vi "Clone.vi"(8 "Error In":errorcluster, 11 "reference in":refnum<class "Rectangle.lvclass">) -> (0 "Error Out":errorcluster, 2 "Return(LabVIEW Object)":refnum<class "ICloneable.lvclass">, 3 "reference out":refnum<class "Rectangle.lvclass">)   [LabVIEW 2020, in "Rectangle.lvclass"]
uses:
  Rectangle.lvclass
  C:/Projects/DesignPatterns/PrototypePattern/ICloneable_interface/ICloneable.lvclass
  ICloneable_interface/ICloneable.lvclass
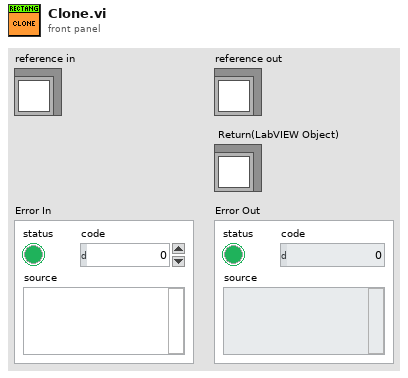
[diagram p1: front panel]
types:
  T1 = typedef "Rectangle.lvclass/ObjectAttributes.ctl" = cluster{"_width":i32, "_height":i32}
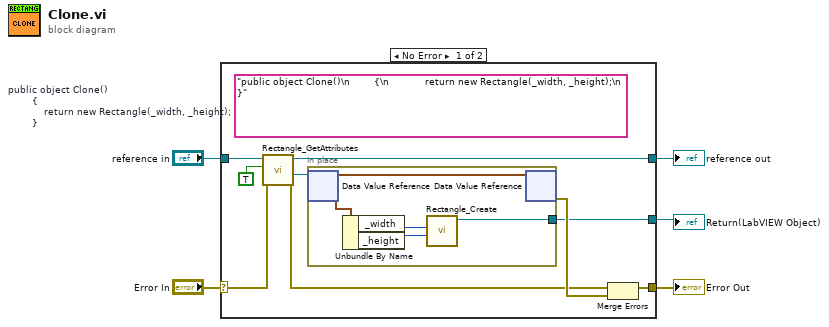
[diagram p0: block diagram]
diagram:
  n1 = case shown="No Error" "Error In" {
    selector: "Error In" -> [w13 w20]
    tunnel: [w10 w20] -> w4
    tunnel: [w11 w19] -> w2
    tunnel: "reference in" -> [w14 w19]
    tunnel: [w6 _] -> w1
    frame No Error {
      (unwired) "public object Clone()\n        {\n            return new Rectangle(_width, _height);\n        }"  # public object Clone()         {             return new Rectangle(_width, _height);         }
      n2 = call "Rectangle_GetAttributes.vi"("error in (no error)"=w13, "OnlyGetDvrReference(False)"=TRUE, "reference in"=w14) -> ("error out"=w8:errorcluster, "DataRef"=w9:refnum<data-value>, "reference out"=w11:refnum<class "Rectangle.lvclass">)  [unwired: 5 in, 1 out]
      n3 = in-place {
        in-place-border: [w16] -> w6
        n4 = in-place-dvr #1(w9) -> (w15:T1)  [unwired: 1 out]
        n5 = Unbundle By Name(w15) -> ("_width"=w17:i32, "_height"=w18:i32)
        n6 = call "Rectangle_Create.vi"("H"=w18, "W"=w17) -> ("reference out"=w16:refnum<class "Rectangle.lvclass">)  [unwired: 8 in, 1 out]
        n7 = in-place-dvr #1(w15) -> (w12:errorcluster)  [unwired: 1 out]
      }
      n8 = Merge Errors(w8, w12) -> (w10:errorcluster)
    }
    frame Error {
    }
  }
  "Error Out" <- w4
  "reference out" <- w2
  "Return(LabVIEW Object)" <- w1
